vi "Exercise 4.2 - Creating a Sub VI.vi"(0 "x":dbl, 1 "y":dbl) -> (7 "x+y":dbl)   [LabVIEW 2012]
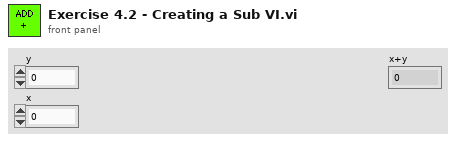
[diagram p1: front panel]
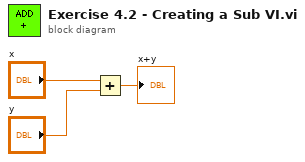
[diagram p0: block diagram]
diagram:
  n1 = Add(x="x", y="y") -> (x+y=→"x+y":dbl)
